vi "Build Text.vi"(10 "angle units":T1, 11 "heading (rad)":dbl) -> (3 "text":string)   [LabVIEW 2017, in "NI_Robotics_Compass Picture.lvlib"]
uses:
  <vilib>/robotics/Controls/Compass Indicator/Compass Picture/NI_Robotics_Compass Picture.lvlib
  <vilib>/robotics/Controls/Utilities/Angle Units.ctl
  <vilib>/Utility/AngleManip/Radians to Degrees (Scalar DBL).vi
  <vilib>/Utility/AngleManip/NI_AngleManipulation.lvlib
  <vilib>/robotics/Controls/Utilities/NI_Robotics_Control Utilities.lvlib
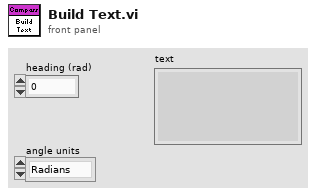
[diagram p1: front panel]
types:
  T1 = typedef "NI_Robotics_Control Utilities.lvlib/Angle Units.ctl" = enum16{"Radians", "Degrees"}
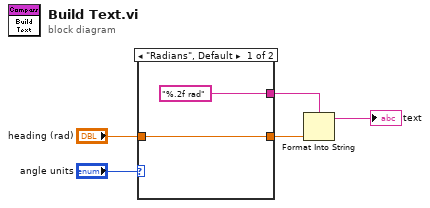
[diagram p0: block diagram]
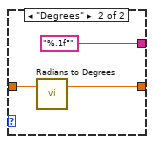
[diagram p2: hidden frame]
diagram:
  n1 = case shown="\"Radians\", Default" "angle units" {
    tunnel: "heading (rad)" -> [w7 w10]
    tunnel: [w7 w9] -> w3
    tunnel: ["%.2f rad" ("format string") "%.1f°" ("format string")] -> w1
    frame "Radians", Default {
    }
    frame "Degrees" {
      n2 = call-poly <vilib>:"Radians to Degrees.vi"("angle (rad)"=w10) -> ("angle (deg)"=w9:dbl)  [unwired: 2 in]
    }
  }
  n3 = Format Into String(format string=w1, w3) -> (resulting string=→"text":string)  [unwired: 2 in, 1 out]
